vi "SetPPMSTemp.vi"(0 "Type":dbl, 1 "Rate":dbl=10.0, 2 "Temp":dbl=300.0) -> ()   [LabVIEW 2013]
uses:
  C:/QdLabview/QDInstrument.dll
panel:
  in  "Instrument\nType 2":i32(ring) items=["PPMS", "VersaLab", "DynaCool", "SVSM"]
  in  "Remote 2":bool
  in  "IP Address 2":string="127.0.0.1"
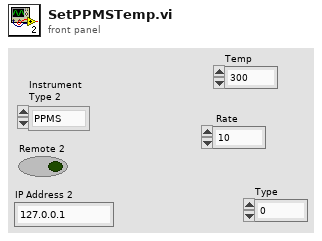
[diagram p1: front panel]
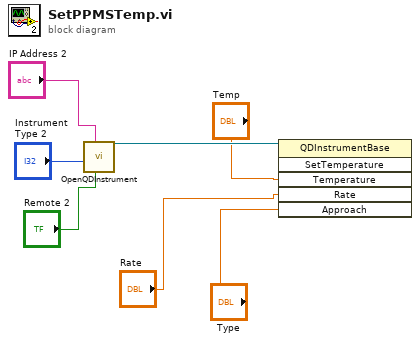
[diagram p0: block diagram]
diagram:
  n1 = call "OpenQDInstrument.vi"("Remote"="Remote 2", "IP Address"="IP Address 2", "Instrument Type"="Instrument\nType 2") -> ("Instrument Ref"=w4:refnum<k24>)  [unwired: 5 in, 1 out]
  n2 = invoke class="QDInstrumentBase" method="SetTemperature"(reference=w4, "Temperature"="Temp", "Rate"="Rate", "Approach"="Type") -> ()  [unwired: 2 in, 6 out]
